vi "MS Read U.vi"(8 "error in (no error)":errorcluster, 9 "U (def. przysp)":enum16{"U przysp", "U jon"}(ring), 10 "delay (ms)":u32=40, 11 "VISA Refnum in":refnum<visa-resource-name>) -> (0 "error out":errorcluster, 1 "Napiecie":dbl, 2 "read buffer":string, 3 "VISA Refnum out":refnum<visa-resource-name>)   [LabVIEW 2012]
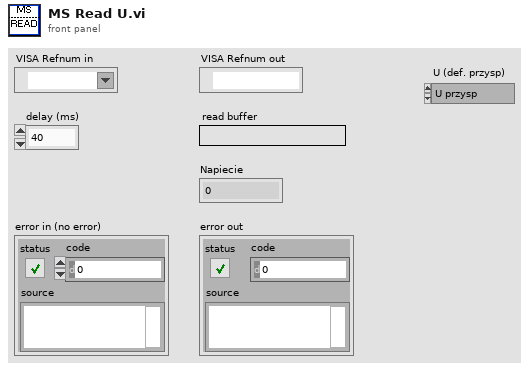
[diagram p1: front panel]
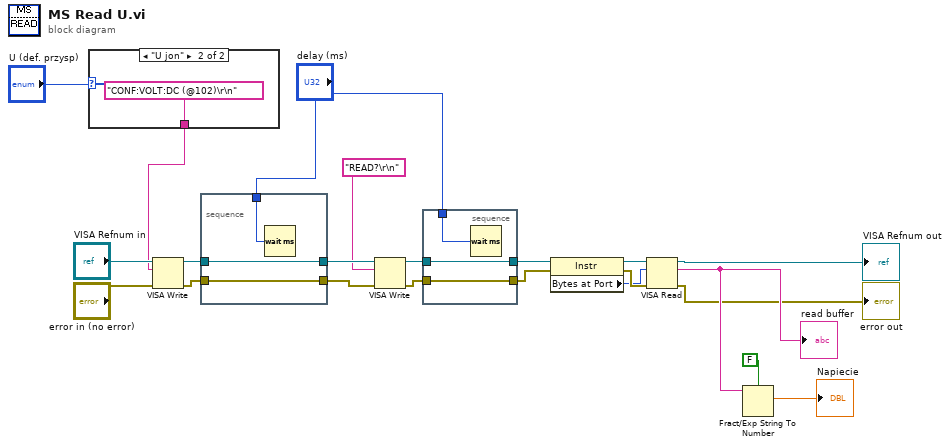
[diagram p0: block diagram]
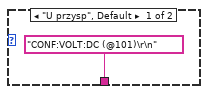
[diagram p2: hidden frame]
diagram:
  n1 = case shown="\"U jon\"" "U (def. przysp)" {
    tunnel: ["CONF:VOLT:DC (@101)\r\n" ("write buffer") "CONF:VOLT:DC (@102)\r\n" ("write buffer")] -> w1
    frame "U przysp", Default {
    }
    frame "U jon" {
    }
  }
  n2 = VISA Write(VISA resource name="VISA Refnum in", write buffer=w1, error in (no error)="error in (no error)") -> (VISA resource name out=w17:refnum<visa-resource-name>, error out=w18:errorcluster)  [unwired: 1 out]
  n3 = stacked-sequence {
    tunnel: [w27] -> w19
    tunnel: w17 -> [w27]
    tunnel: w18 -> [w26]
    tunnel: [w26] -> w20
    tunnel: "delay (ms)" -> [w25]
    frame #0 {
      n4 = Wait (ms)(milliseconds to wait=w25) -> ()  [unwired: 1 out]
    }
  }
  n5 = VISA Write(VISA resource name=w19, write buffer="READ?\r\n", error in (no error)=w20) -> (VISA resource name out=w12:refnum<visa-resource-name>, error out=w13:errorcluster)  [unwired: 1 out]
  n6 = stacked-sequence {
    tunnel: [w30] -> w11
    tunnel: w12 -> [w30]
    tunnel: w13 -> [w29]
    tunnel: [w29] -> w14
    tunnel: "delay (ms)" -> [w28]
    frame #0 {
      n7 = Wait (ms)(milliseconds to wait=w28) -> ()  [unwired: 1 out]
    }
  }
  n8 = property class="Instr"(reference=w11, error in=w14) -> (reference out=w7:refnum<visa-resource-name>, error out=w8:errorcluster, "Bytes at Port"=w6:u32)
  n9 = VISA Read(VISA resource name=w7, byte count=w6, error in (no error)=w8) -> (VISA resource name out=→"VISA Refnum out":refnum<visa-resource-name>, read buffer=w15:string, error out=→"error out":errorcluster)  [unwired: 1 out]
  "read buffer" <- w15
  n10 = Fract/Exp String To Number(use system decimal point (T)=FALSE, string=w15) -> (number=→"Napiecie":dbl)  [unwired: 2 in, 1 out]
